vi "Material-Line2-Aquisition.vi"(8 "error in (no error)":errorcluster, 11 "Material-RunTest in":refnum<class "Material-RunTest.lvclass">) -> (0 "error out":errorcluster, 3 "Material-RunTest out":refnum<class "Material-RunTest.lvclass">)   [LabVIEW 2013, in "Material-RunTest.lvclass"]
uses:
  Material-RunTest.lvclass
  Material-RunTest.lvclass/Material-RunTest.ctl
  <instrlib>/Keyence LK-G5000/Public/enum/LKIF_OUTNO.ctl
  <instrlib>/Keyence LK-G5000/Keyence LK-G5000.lvlib
  Motion Control/Motion-ControlAll.lvclass
panel:
  out "Laser Value":sgl format="%_6g"
  out "Init Meas1":dbl[](array[numeric])
  out "stop collecting":bool
  out "Meas 1 Dyn Data":dbl[](graph)
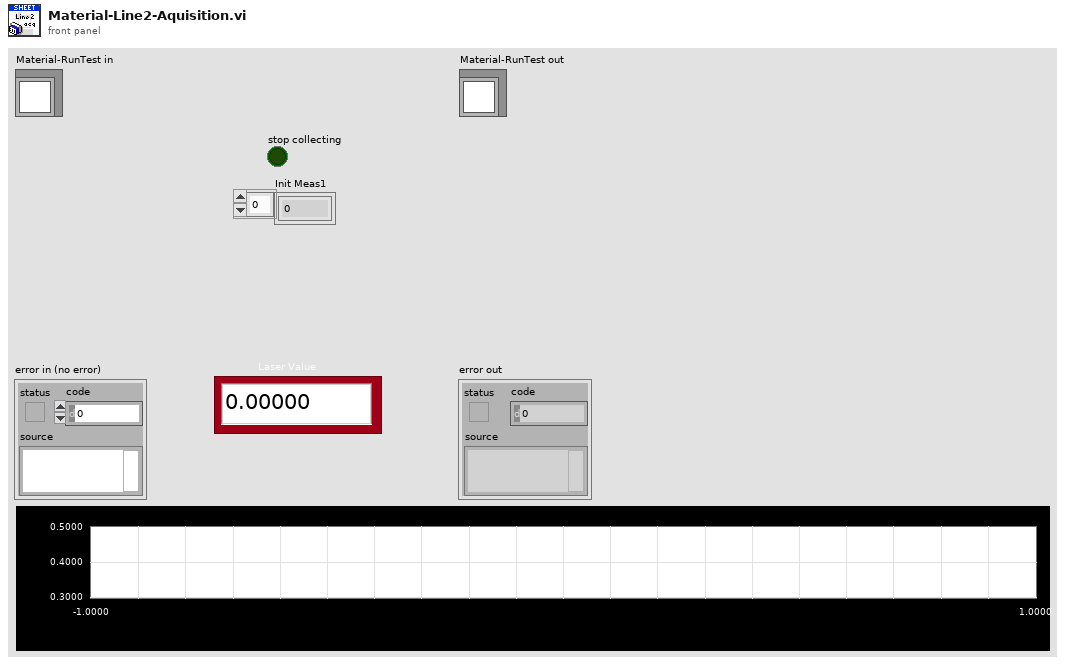
[diagram p1: front panel]
types:
  T1 = typedef "Keyence LK-G5000.lvlib/LKIF_OUTNO.ctl" = i32
  T2 = typedef "Keyence LK-G5000.lvlib/LKIF_FLOATRESULT.ctl" = i32
  T3 = cluster{"OutNo":i32, "LKIF_FLOATRESULT":T2, "Value":sgl}[]
  T4 = cluster{"OutNo":i32, "LKIF_FLOATRESULT":T2, "Value":sgl}
  T5 = cluster{waveform(dbl), waveform(dbl), waveform(dbl)}
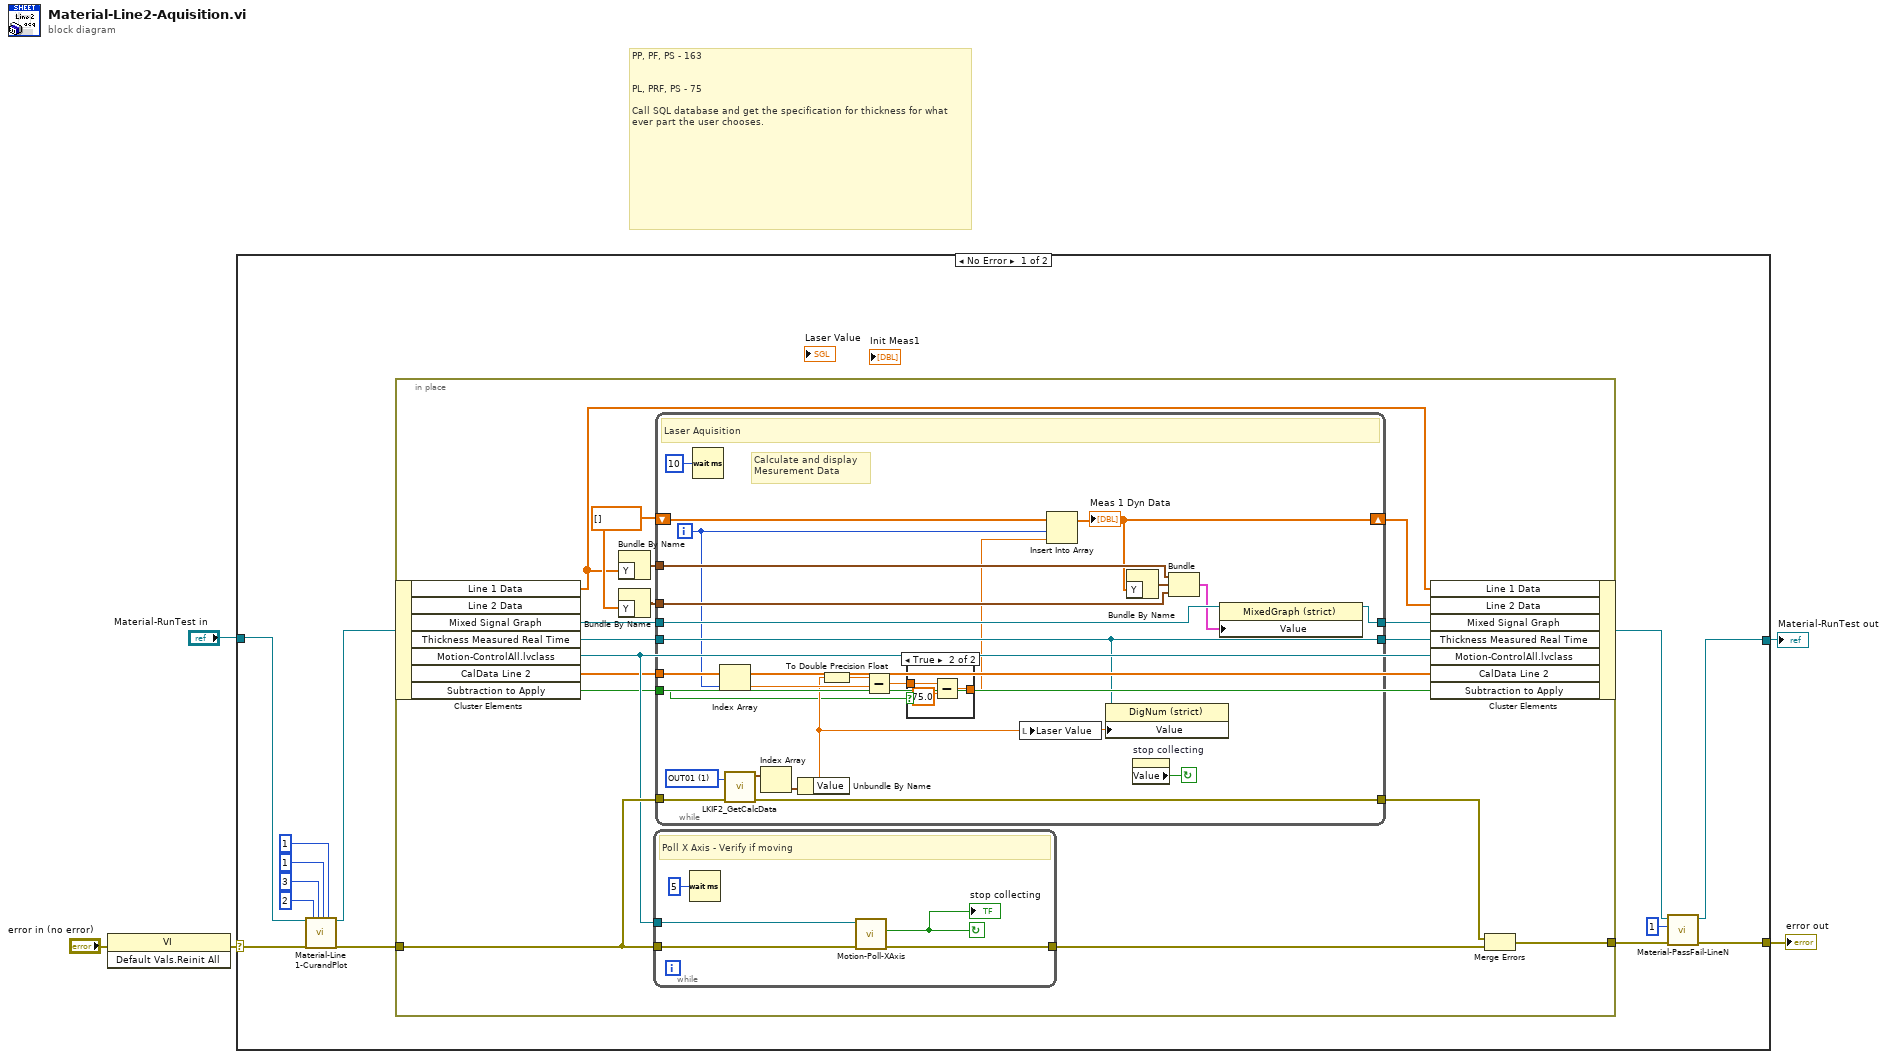
[diagram p0: block diagram]
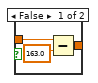
[diagram p2: hidden frame]
diagram:
  # "PP, PF, PS - 163\n\n\nPL, PRF, PS - 75\n\nCall SQL database and get the specification for thickness for what ever part the user chooses."
  n1 = invoke class="VI" method="Default Vals.Reinit All"(error in="error in (no error)") -> (error out=w1:errorcluster)  [unwired: 2 in, 2 out]
  n2 = case shown="No Error" w1 {
    selector: w1 -> [w13 w71]
    tunnel: [w6 w71] -> w5
    tunnel: [w7 w70] -> w3
    tunnel: "Material-RunTest in" -> [w18 w70]
    frame No Error {
      n3 = call "Material-Line 1-CurandPlot.vi"("Material-RunTest in"=w18, "error in (no error)"=w13, "Active Cursor Max"=u32 2, "Active Cursor Min"=u32 3, "Active Y Scale"=1, "Active Plot"=u32 1) -> ("Material-RunTest out"=w11:refnum<class "Material-RunTest.lvclass">, "error out"=w12:errorcluster)  [unwired: 12 in]
      n4 = in-place {
        in-place-border: w12 -> [w34]
        in-place-border: [w26] -> w10
        w23 = dbl[] []
        n5 = in-place-cluster #1(w11) -> ("Line 1 Data"=w21:dbl[], "Mixed Signal Graph"=w32:refnum<vi>, "Thickness Measured Real Time"=w33:refnum<vi>, "Motion-ControlAll.lvclass"=w29:refnum<class "Motion-ControlAll.lvclass">, "CalData Line 2"=w20:dbl[], "Subtraction to Apply"=w19:bool)  [unwired: 1 out]
        n6 = Bundle By Name("Y"=w21) -> (w24:waveform(dbl))  [unwired: 1 in]
        n7 = Bundle By Name("Y"=w23) -> (w22:waveform(dbl))  [unwired: 1 in]
        n8 = while {
          tunnel: w34 -> [w38]
          tunnel: [w36] -> w28
          tunnel: w29 -> [w37]
          stop <- w35 continue-if-true
          # "Poll X Axis - Verify if moving"
          n9 = Wait (ms)(milliseconds to wait=u32 5) -> ()  [unwired: 1 out]
          n10 = call "Motion-Poll-XAxis.vi"("error in (no error)"=w38, "Motion-ControlAll in"=w37) -> ("error out"=w36:errorcluster, "X axis \nstopped"=w35:bool)  [unwired: 7 in, 1 out]
          "stop collecting" <- w35
        }
        n11 = while {
          tunnel: w34 -> [w63]
          tunnel: [w59] -> w27
          tunnel: w33 -> [w54]
          shift-right: [w50] -> w25
          shift-left: w23 -> [w57]
          tunnel: w32 -> [w56]
          tunnel: [w55] -> w31
          tunnel: [w54] -> w30
          tunnel: w24 -> [w52]
          tunnel: w22 -> [w51]
          tunnel: w20 -> [w49]
          tunnel: w19 -> [w43]
          i -> [w48]
          stop <- w53 continue-if-true
          w62 = T1 1 items=["OUT01"=1, "OUT02"=2, "OUT03"=4, "OUT04"=8, "OUT05"=16, "OUT06"=32, "OUT07"=64, "OUT08"=128, "OUT09"=256, "OUT10"=512, "OUT11"=1024, "OUT12"=2048, "ALL OUT"=4095] ("OutNo (OUT1)")
          # "Calculate and display \nMesurement Data"
          # "Laser Aquisition"
          n12 = Wait (ms)(milliseconds to wait=u32 10) -> ()  [unwired: 1 out]
          n13 = Index Array(array=w49, index=w48) -> (element=w47:dbl)
          n14 = call <instrlib>:"LKIF2_GetCalcData.vi"("OutNo (OUT1)"=w62, "error in (no error)"=w63) -> ("error out"=w59:errorcluster, "CalcData"=w61:T3)  [unwired: 8 in]
          n15 = Index Array(array=w61) -> (element=w60:T4)  [unwired: 1 in]
          n16 = Unbundle By Name(w60) -> ("Value"=w46:sgl)
          n17 = To Double Precision Float(number=w46) -> (double precision float=w45:dbl)
          n18 = Subtract(x=w45, y=w47) -> (x-y=w44:dbl)
          n19 = case shown="True" w43 {
            tunnel: w44 -> [w65 w69]
            tunnel: [w64 w67] -> w42
            frame False {
              n20 = Subtract(x=w65, y=163.0) -> (x-y=w64:dbl)
            }
            frame True {
              n21 = Subtract(x=w69, y=75.0) -> (x-y=w67:dbl)
            }
          }
          n22 = local write "Laser Value"(w46) -> ()
          n23 = Insert Into Array(array=w57, index=w48, new element=w42) -> (w50:dbl[])
          "Meas 1 Dyn Data" <- w50
          n24 = property class="DigNum (strict)"(reference=w54, "Value"=w46) -> ()  [unwired: 1 in, 2 out]
          n25 = Bundle By Name("Y"=w50) -> (w41:waveform(dbl))  [unwired: 1 in]
          n26 = property on="stop collecting" class="Bool (strict)"() -> ("Value"=w53:bool)  [unwired: 2 in, 2 out]
          n27 = Bundle(w52, w41, w51) -> (w40:T5)  [unwired: 1 in]
          n28 = property class="MixedGraph (strict)"(reference=w56, "Value"=w40) -> (reference out=w55:refnum<vi>)  [unwired: 1 in, 1 out]
        }
        n29 = in-place-cluster #1("Line 1 Data"=w21, "Line 2 Data"=w25, "Mixed Signal Graph"=w31, "Thickness Measured Real Time"=w30, "Motion-ControlAll.lvclass"=w29, "CalData Line 2"=w20, "Subtraction to Apply"=w19) -> (w9:refnum<class "Material-RunTest.lvclass">)
        n30 = Merge Errors(w27, w28) -> (w26:errorcluster)
      }
      n31 = call "Material-PassFail-LineN.vi"("error in (no error)"=w10, "Line?"=1, "Material-RunTest in"=w9) -> ("error out"=w6:errorcluster, "Material-RunTest out"=w7:refnum<class "Material-RunTest.lvclass">)  [unwired: 7 in]
    }
    frame Error {
    }
  }
  "error out" <- w5
  "Material-RunTest out" <- w3
